vi "prompt user for json file location.vi"(8 "error in":errorcluster) -> (0 "error out":errorcluster, 2 "cancelled":bool, 3 "selected path":path)   [LabVIEW 2020]
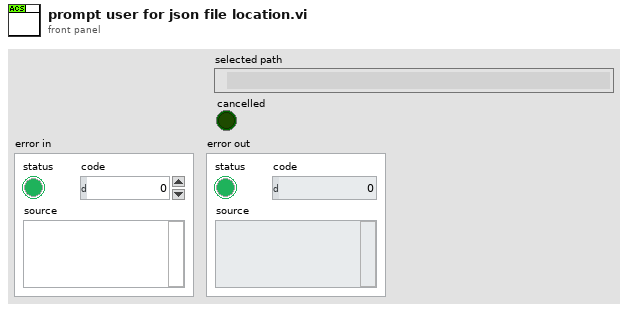
[diagram p1: front panel]
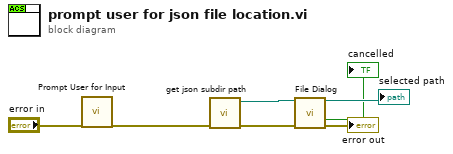
[diagram p0: block diagram]
diagram:
  n1 = call "Prompt User for Input"("error in (no error)"="error in") -> ("error out"=w6:errorcluster)  [unwired: 17 in, 1 out]
  n2 = call "get json subdir path.vi"("error in"=w6) -> ("error out"=w5:errorcluster, "json path"=w7:path)  [unwired: 9 in]
  n3 = call "File Dialog"("start path"=w7, "error in"=w5) -> ("selected path"=→"selected path":path, "cancelled"=→"cancelled":bool, "error out"=→"error out":errorcluster)  [unwired: 10 in, 1 out]
